vi "SubVI_Set_37_arm.vi"(8 "error in (no error)":errorcluster, 11 "TCP Network Connection in":refnum<k5>) -> (0 "error out":errorcluster, 3 "TCP Network Connection out":refnum<k5>)   [LabVIEW 2020]
panel:
  out "data out":string
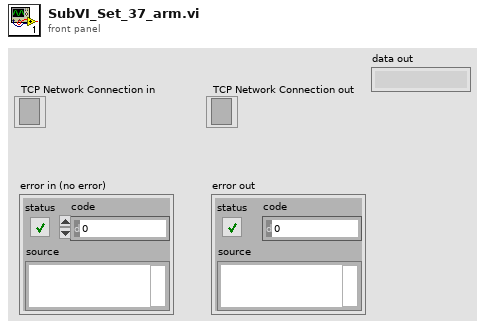
[diagram p1: front panel]
types:
  T1 = enum16{"Standard", "Buffered", "CRLF", "Immediate"}
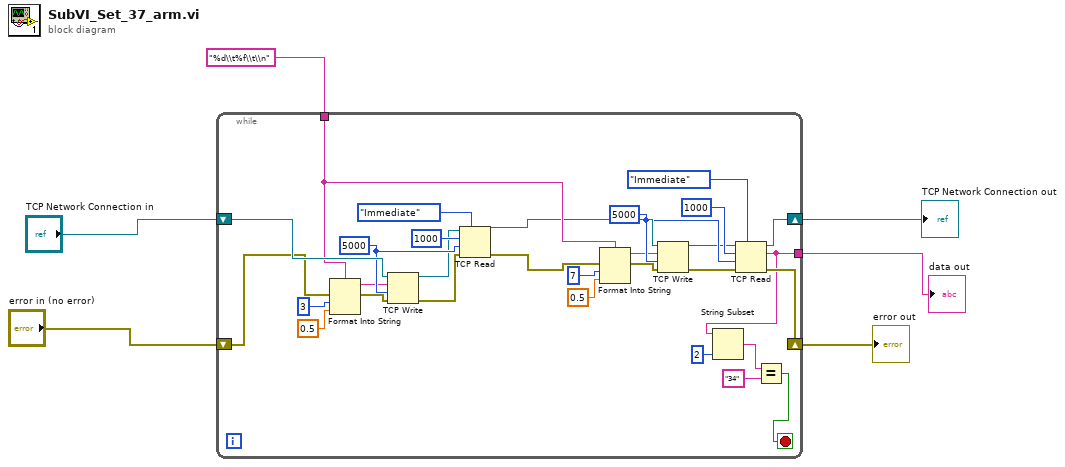
[diagram p0: block diagram]
diagram:
  n1 = while {
    tunnel: "%d\\t%f\\t\\n" ("format string") -> [w32]
    tunnel: [w11] -> w1
    shift-right: [w36] -> w6
    shift-left: "TCP Network Connection in" -> [w34]
    shift-right: [w35] -> w5
    shift-left: "error in (no error)" -> [w33]
    stop <- w7 stop-if-true
    w20 = 5000 ("timeout ms (25000)")
    w29 = 5000 ("timeout ms (25000)")
    n2 = Format Into String(format string=w32, error in=w33, 3 ("input 1"), 0.5) -> (resulting string=w14:string, error out=w15:errorcluster)  [unwired: 1 in]
    n3 = TCP Write(connection ID=w34, data in=w14, error in (no error)=w15, 9:w20) -> (connection ID out=w17:refnum<k5>, error out=w16:errorcluster)  [unwired: 1 out]
    n4 = TCP Read(connection ID=w17, bytes to read=1000, error in (no error)=w16, 7:T1."Immediate" ("mode (standard)"), 9:w20) -> (connection ID out=w31:refnum<k5>, error out=w30:errorcluster)  [unwired: 1 out]
    n5 = Format Into String(format string=w32, error in=w30, 7 ("input 1"), 0.5) -> (resulting string=w23:string, error out=w24:errorcluster)  [unwired: 1 in]
    n6 = TCP Write(connection ID=w31, data in=w23, error in (no error)=w24, 9:w29) -> (connection ID out=w26:refnum<k5>, error out=w25:errorcluster)  [unwired: 1 out]
    n7 = TCP Read(connection ID=w26, bytes to read=1000, error in (no error)=w25, 7:T1."Immediate" ("mode (standard)"), 9:w29) -> (connection ID out=w36:refnum<k5>, data out=w11:string, error out=w35:errorcluster)
    n8 = String Subset(string=w11, length (rest)=2 ("length (rest)")) -> (substring=w9:string)  [unwired: 1 in]
    n9 = Equal?(x=w9, y="34") -> (x = y?=w7:bool)
  }
  "TCP Network Connection out" <- w6
  "error out" <- w5
  "data out" <- w1
